vi "Stage2Lambda.vi"(4 "intercept":dbl, 6 "slope":dbl, 11 "Stage (mm)":dbl) -> (3 "lambda":dbl)   [LabVIEW 2025]
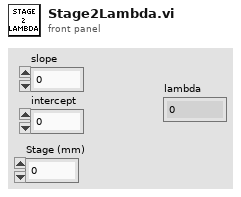
[diagram p1: front panel]
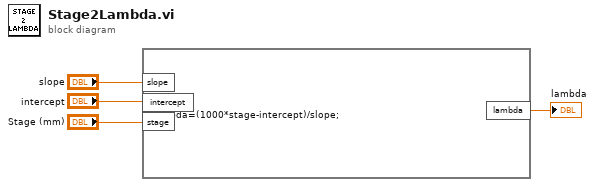
[diagram p0: block diagram]
diagram:
  n1 = formula code="lambda=(1000*stage-intercept)/slope;"("slope"="slope", "intercept"="intercept", "stage"="Stage (mm)") -> ("lambda"=→"lambda":dbl)
